vi "MercuryITC-VISA-read.vi"(8 "error in (no error)":errorcluster, 10 "write buffer":string, 11 "VISA resource name":refnum<visa-resource-name>) -> (0 "error out":errorcluster, 2 "read buffer":string, 3 "VISA resource name out":refnum<visa-resource-name>)   [LabVIEW 2012]
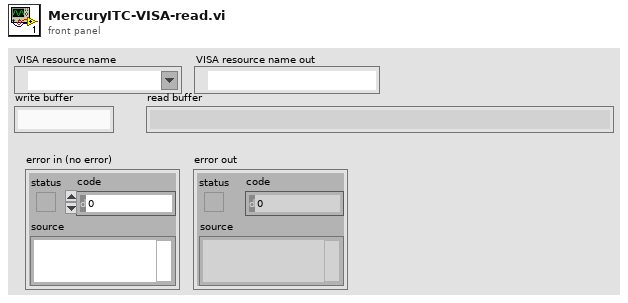
[diagram p1: front panel]
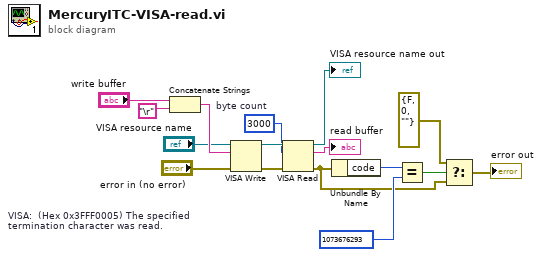
[diagram p0: block diagram]
diagram:
  w7 = 1073676293  # VISA:  (Hex 0x3FFF0005) The specified termination character was read.
  w14 = u32 3000  # byte count
  n1 = Concatenate Strings("write buffer", "\r") -> (w10:string)
  n2 = VISA Write(VISA resource name="VISA resource name", write buffer=w10, error in (no error)="error in (no error)") -> (VISA resource name out=w15:refnum<visa-resource-name>, error out=w16:errorcluster)  [unwired: 1 out]
  n3 = VISA Read(VISA resource name=w15, byte count=w14, error in (no error)=w16) -> (VISA resource name out=→"VISA resource name out":refnum<visa-resource-name>, read buffer=→"read buffer":string, error out=w5:errorcluster)  [unwired: 1 out]
  n4 = Unbundle By Name(w5) -> ("code"=w8:i32)
  n5 = Equal?(x=w8, y=w7) -> (x = y?=w4:bool)
  n6 = Select(t=errorcluster {"status"=FALSE, "code"=0, "source"=""}, s=w4, f=w5) -> (s? t:f=→"error out":errorcluster)
